vi "HDF5_Init_Filter_Refs.vi"(5 "HDF5 file ref":T2 format="%.0x", 9 "File Exists?":bool, 11 "error in":errorcluster) -> (4 "Filter_Refs":T1 {"Filter_Group_ref" format="%.0x"; "TimeStamp_dset" format="%.0x"; "Filter_dset" format="%.0x"}, 6 "HDF5 file ref":T2 format="%.0x", 15 "error out":errorcluster)   [LabVIEW 2018]
doc: "Set up the HDF5 data structure and initialize the references for the Tone1, Tone2, Tone3, and Tone4 Groups and the datasets (tables) within each Group.\n\nData structure:\nTone1 (Group) \n Beac - cluster (Dataset)\n BeacZoom - 1024 element Double array (waveform) \n Cal - cluster\n CalZoom - 1024 element Double array (waveform) \nTone2\n Beac - cluster\n BeacZoom - 1024 element Double array (waveform) \n Cal - cluster\n CalZoom - 1024 element Double array (waveform) \nTone3\n Beac - cluster\n BeacZoom - 1024 element Double array (waveform) \n Cal - cluster\n CalZoom - 1024 element Double array (waveform) \nTone4\n Beac - cluster\n BeacZoom - 1024 element Double array (waveform) \n Cal - cluster\n CalZoom - 1024 element Double array (waveform)"
uses:
  <vilib>/addons/h5labview2/base/hid_t.ctl
  HDF5_Filter_refs.ctl
  lib_path_mod_20200519.vi
  <vilib>/addons/h5labview2/base/H5Equery.vi
  <vilib>/addons/h5labview2/attrib/H5Awrite.llb/H5Awrite.xnode
  <vilib>/addons/h5labview2/group/H5G.lvlib
  <vilib>/addons/h5labview2/dataset/H5D.lvlib
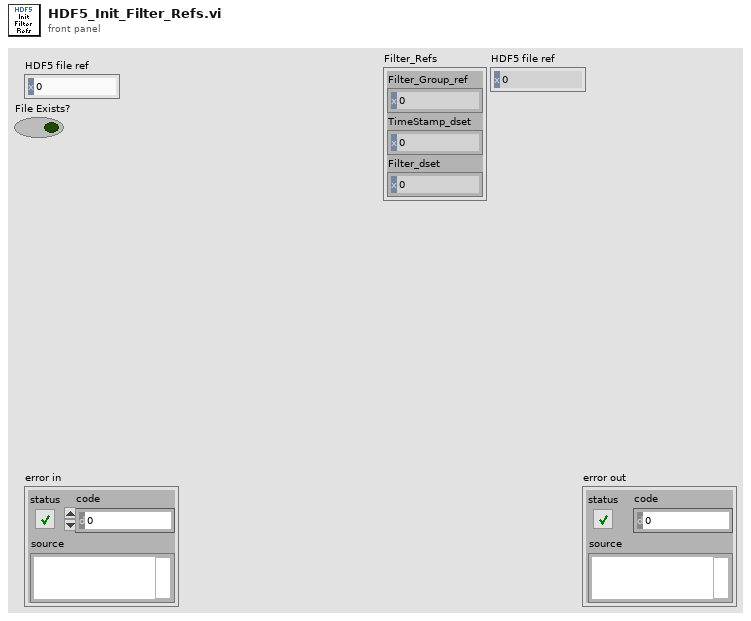
[diagram p1: front panel]
types:
  T1 = typedef "HDF5_Filter_refs.ctl" = cluster{"Filter_Group_ref":T2, "TimeStamp_dset":T2, "Filter_dset":T2}
  T2 = typedef "hid_t.ctl" = i32
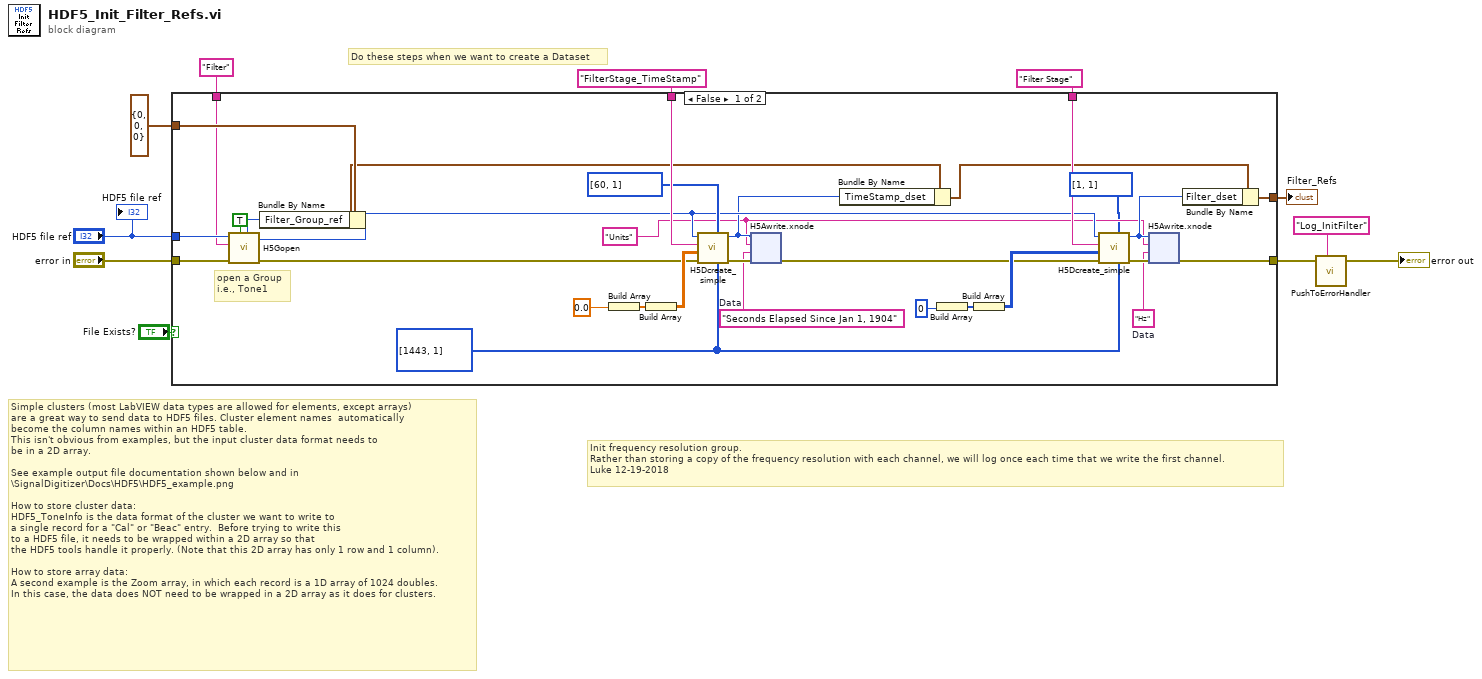
[diagram p0: block diagram]
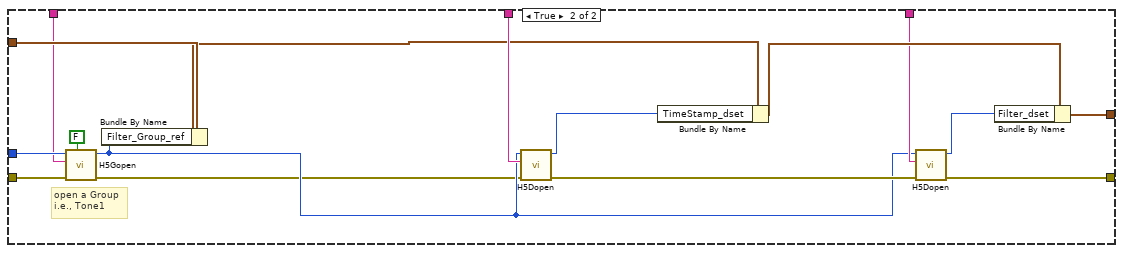
[diagram p2: hidden frame]
diagram:
  # "Init frequency resolution group.\nRather than storing a copy of the frequency resolution with each channel, we will log once each time that we write the first channel.\nLuke 12-19-2018"
  # "Do these steps when we want to create a Dataset"
  # "Simple clusters (most LabVIEW data types are allowed for elements, except arrays) \nare a great way to send data to HDF5 files. Cluster element names  automatically\nbecome the column names within an HDF5 table.\nThis isn't obvious from examples, but the input cluster data format needs to \nbe in a 2D array.\n\nSee example output file documentation shown below and in\n\\SignalDigitizer\\Docs\\HDF5\\HDF5_example.png\n\nHow to store cluster data:\nHDF5_ToneInfo is the data format of the cluster we want to write to \na single record for a \"Cal\" or \"Beac\" entry.  Before trying to write this \nto a HDF5 file, it needs to be wrapped within a 2D array so that \nthe HDF5 tools handle it properly. (Note that this 2D array has only 1 row and 1 column).\n\nHow to store array data:\nA second example is the Zoom array, in which each record is a 1D array of 1024 doubles.\nIn this case, the data does NOT need to be wrapped in a 2D array as it does for clusters."
  n1 = case shown="False" "File Exists?" {
    tunnel: "error in" -> [w41 w95]
    tunnel: "HDF5 file ref" -> [w40 w94]
    tunnel: [w13 w81] -> w3
    tunnel: T1 {"Filter_Group_ref"=0, "TimeStamp_dset"=0, "Filter_dset"=0} ("Cluster") -> [w38 w92]
    tunnel: [w14 w80] -> w4
    tunnel: "FilterStage_TimeStamp" ("string") -> [w37 w90]
    tunnel: "Filter Stage" ("string") -> [w34 w87]
    tunnel: "Filter" ("name") -> [w17 w84]
    frame False {
      w18 = "Hz"  # Data
      w20 = "Seconds Elapsed Since Jan 1, 1904"  # Data
      w19 = "Units" ("attrib name")
      w29 = u64[] [1443, 1] ("max size")
      # "open a Group\ni.e., Tone1"
      n2 = call <vilib>:"H5Gopen.vi"("create? (F)"=TRUE, "error in (no error)"=w41, "name"=w17, "ref in"=w40) -> ("error out"=w16:errorcluster, "group out"=w27:T2)  [unwired: 6 in]
      n3 = Bundle By Name(cluster=w38, "Filter_Group_ref"=w27) -> (w15:T1)
      n4 = Build Array(0.0 ("TimeStamp")) -> (w35:dbl[])
      n5 = Build Array(w35) -> (w36:dbl[][])
      n6 = call <vilib>:"H5Dcreate_simple.vi"("max size"=w29, "chunk size"=u64[] [60, 1], "error in (no error)"=w16, "type in"=w36, "name"=w37, "ref in"=w27) -> ("error out"=w25:errorcluster, "dset out"=w24:T2)  [unwired: 4 in]
      n7 = xnode "H5Awrite.xnode"("error in (no error)"=w25, "data"=w20, "attrib name"=w19, "ref in"=w24) -> ("error out"=w21:errorcluster)  [unwired: 3 in, 2 out]
      n8 = Bundle By Name(cluster=w15, "TimeStamp_dset"=w24) -> (w26:T1)
      n9 = Build Array(u8 0) -> (w32:u8[])
      n10 = Build Array(w32) -> (w33:u8[][])
      n11 = call <vilib>:"H5Dcreate_simple.vi"("max size"=w29, "chunk size"=u64[] [1, 1], "error in (no error)"=w21, "type in"=w33, "name"=w34, "ref in"=w27) -> ("error out"=w22:errorcluster, "dset out"=w23:T2)  [unwired: 4 in]
      n12 = xnode "H5Awrite.xnode"("error in (no error)"=w22, "data"=w18, "attrib name"=w19, "ref in"=w23) -> ("error out"=w13:errorcluster)  [unwired: 3 in, 2 out]
      n13 = Bundle By Name(cluster=w26, "Filter_dset"=w23) -> (w14:T1)
    }
    frame True {
      # "open a Group\ni.e., Tone1"
      n14 = call <vilib>:"H5Gopen.vi"("create? (F)"=FALSE, "error in (no error)"=w95, "name"=w84, "ref in"=w94) -> ("error out"=w82:errorcluster, "group out"=w85:T2)  [unwired: 6 in]
      n15 = Bundle By Name(cluster=w92, "Filter_Group_ref"=w85) -> (w83:T1)
      n16 = call <vilib>:"H5Dopen.vi"("error in (no error)"=w82, "name"=w90, "loc in"=w85) -> ("error out"=w86:errorcluster, "dset out"=w91:T2)  [unwired: 7 in]
      n17 = Bundle By Name(cluster=w83, "TimeStamp_dset"=w91) -> (w88:T1)
      n18 = call <vilib>:"H5Dopen.vi"("error in (no error)"=w86, "name"=w87, "loc in"=w85) -> ("error out"=w81:errorcluster, "dset out"=w89:T2)  [unwired: 7 in]
      n19 = Bundle By Name(cluster=w88, "Filter_dset"=w89) -> (w80:T1)
    }
  }
  "Filter_Refs" <- w4
  n20 = call "PushToErrorHandler.vi"("ErrorIn"=w3, "ErrorLocation"="Log_InitFilter") -> ("ErrorOut"=→"error out":errorcluster)  [unwired: 5 in]
  "HDF5 file ref" <- "HDF5 file ref"
